vi "IDS_Connect.vi"(8 "error in (no error)":errorcluster, 10 "port":i32, 11 "ipAddress":string) -> (0 "error out":errorcluster, 3 "deviceHandle out":i32)   [LabVIEW 2016]
doc: "int IDS_DLL IDS_Connect(char* ipAddress, int port);"
panel:
  out "ipAddress out":string
  out "function return":i32
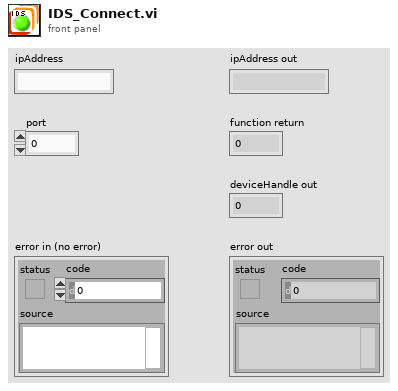
[diagram p1: front panel]
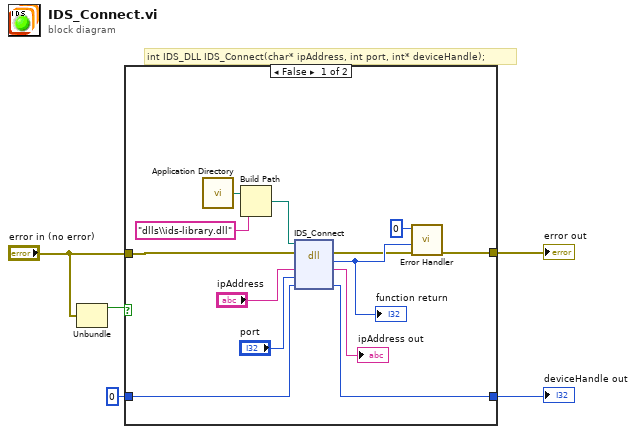
[diagram p0: block diagram]
diagram:
  # "int IDS_DLL IDS_Connect(char* ipAddress, int port, int* deviceHandle);"
  n1 = Unbundle("error in (no error)") -> ("status"=w1:bool)  [unwired: 2 out]
  n2 = case shown="False" w1 {
    tunnel: "error in (no error)" -> [w15 w20]
    tunnel: [w11 w20] -> w5
    tunnel: 0 ("deviceHandle") -> [w14 w19]
    tunnel: [w13 w19] -> w3
    frame False {
      n3 = call <vilib>:"Application Directory.vi"() -> ("Application Directory"=w8:path)
      n4 = Build Path(base path=w8, name or relative path="dlls\\ids-library.dll" ("ipAddress")) -> (appended path=w6:path)
      n5 = dll-call lib="?" fn="IDS_Connect"(path in=w6, error in=w15, "ipAddress"="ipAddress", "port"="port", "deviceHandle"=w14) -> (error out=w10:errorcluster, "return type"=w12:i32, "ipAddress"=→"ipAddress out":string, "deviceHandle"=w13:i32)  [unwired: 2 in, 1 out]
      "function return" <- w12
      n6 = call "Error Handler.vi"("error in (no error)"=w10, "error code"=w12, "deviceHandle"=0) -> ("error out"=w11:errorcluster)  [unwired: 7 in, 1 out]
    }
    frame True {
    }
  }
  "error out" <- w5
  "deviceHandle out" <- w3
